vi "genRVCtraj.vi"() -> ()   [LabVIEW 2016]
uses:
  <vilib>/Math Plots/3D Math Plots/3D Scatter/3D Scatter XCtrl/3D Scatter.xctl
  <vilib>/Analysis/1siggen.llb/Ramp Pattern by Samples.vi
  <vilib>/Utility/file.llb/Read Delimited Spreadsheet (DBL).vi
  Subsystems/Global Variables.vi
  <vilib>/Math Plots/3D Math Plots/3D Scatter/3D Scatter Datatype/Public/Plot Helper (Vector).vi
  <vilib>/Math Plots/3D Math Plots/3D Scatter/3D Scatter Datatype/3D Scatter Datatype.lvclass
  <vilib>/gmath/NI_Gmath.lvlib
  <vilib>/Analysis/NI_AALBase.lvlib
panel:
  out "DH Params":cluster{"d_DH":dbl[][], "ty":dbl[][]}
  out "J3 Array":dbl[](array[numeric])
  out "J2 Array":dbl[](array[numeric])
  out "J1 Array":dbl[](array[numeric])
  in  "offsetZ":dbl
  in  "offsetX":dbl
  in  "offsetY":dbl
  out "size(s)":i32
  out "zVisTraj":dbl[](array[numeric]) format="%_6g"
  out "yVisTraj":dbl[](array[numeric]) format="%_6g"
  out "xVisTraj":dbl[](array[numeric]) format="%_6g"
  out "Groove Plot":refnum<class "3D Plot Datatype.lvclass">[](xcontrol)
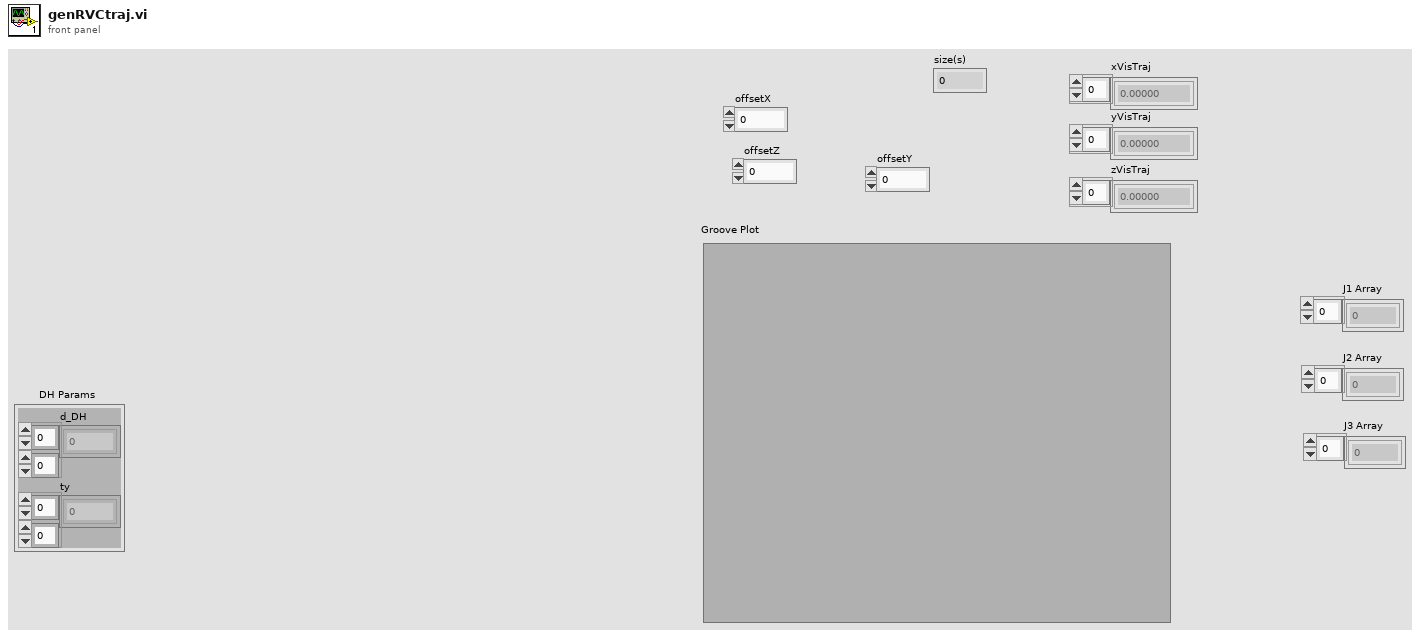
[diagram p1: front panel]
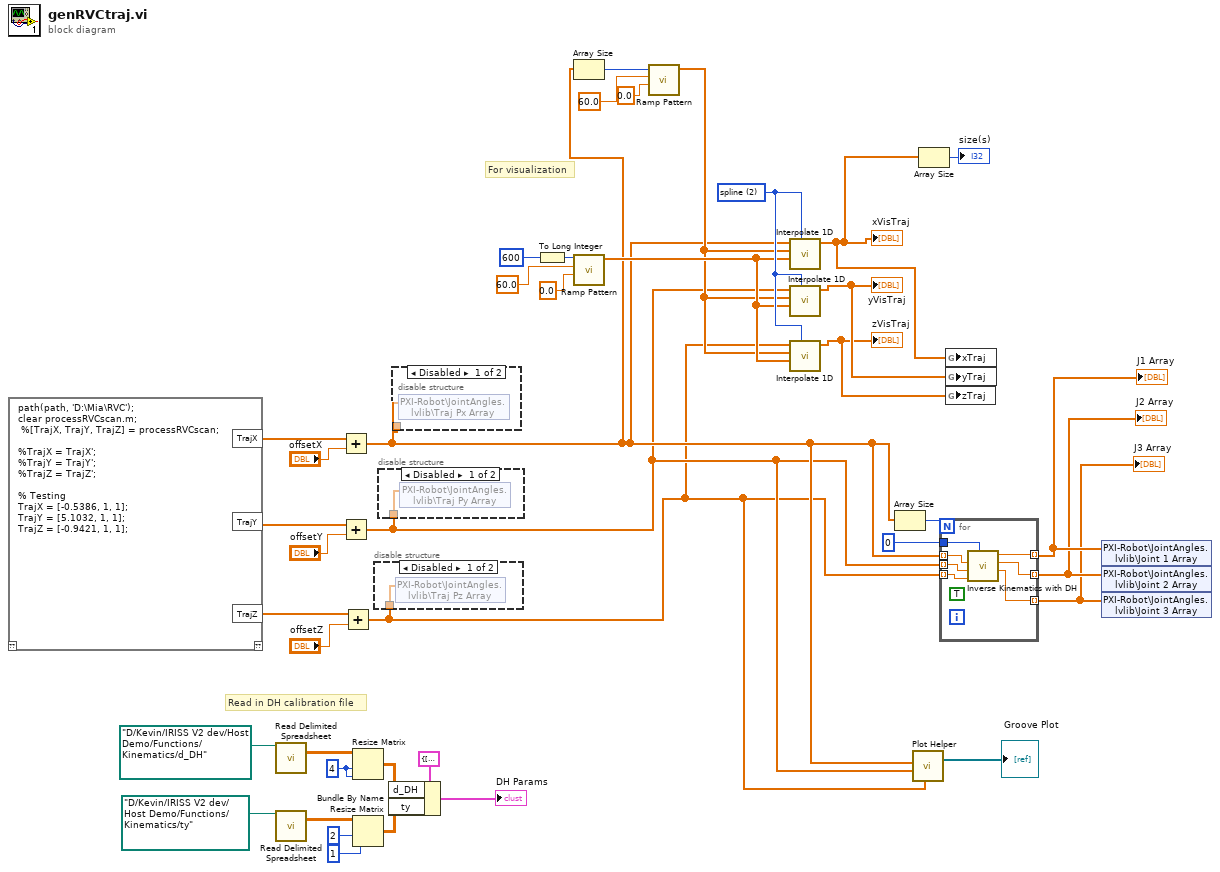
[diagram p0: block diagram]
diagram:
  w9 = 4 ("number of rows")
  w40 = 2 items=["nearest", "linear", "spline", "cubic Hermite", "Lagrange"] ("method")
  # "Read in DH calibration file"
  # "For visualization"
  n1 = script code="path(path, 'D:\\Mia\\RVC'); \nclear processRVCscan.m; \n %[TrajX, TrajY, TrajZ] = processRVCscan; \n\n%TrajX = TrajX'; \n%TrajY = TrajY'; \n%TrajZ = TrajZ'; \n\n% Testing \nTrajX = [-0.5386, 1, 1]; \nTrajY = [5.1032, 1, 1]; \nTrajZ = [-0.9421, 1, 1];"() -> ("TrajX"=w19:dbl[], "TrajY"=w18:dbl[], "TrajZ"=w16:dbl[])  [unwired: 1 in, 1 out]
  n2 = call-poly <vilib>:"Read Delimited Spreadsheet.vi"("file path (dialog if empty)"=path "D:/Kevin/IRISS V2 dev/Host Demo/Functions/Kinematics/d_DH" ("file path (use dialog)")) -> ("all rows"=w10:dbl[][])  [unwired: 9 in, 5 out]
  n3 = call-poly <vilib>:"Read Delimited Spreadsheet.vi"("file path (dialog if empty)"=path "D:/Kevin/IRISS V2 dev/Host Demo/Functions/Kinematics/ty" ("file path (use dialog)")) -> ("all rows"=w8:dbl[][])  [unwired: 9 in, 5 out]
  n4 = Add(x=w19, y="offsetX") -> (x+y=w20:dbl[])
  n5 = Add(x=w18, y="offsetY") -> (x+y=w17:dbl[])
  n6 = Add(x=w16, y="offsetZ") -> (x+y=w15:dbl[])
  n7 = Resize Matrix(1:w9, 2:w9, 4:w10) -> (0:w4:dbl[][])
  n8 = Resize Matrix(1:1 ("number of columns"), 2:2 ("number of rows"), 4:w8) -> (0:w3:dbl[][])
  n9 = disable-structure shown="Disabled" {
    disable-tunnel: w15 -> [w41 _]
    frame Disabled {
      n10 = shared-variable "PXI-Robot\\JointAngles.lvlib\\Traj Pz Array"(w41) -> ()  [unwired: 1 in, 1 out]
    }
    frame Enabled {
    }
  }
  n11 = disable-structure shown="Disabled" {
    disable-tunnel: w17 -> [w42 _]
    frame Disabled {
      n12 = shared-variable "PXI-Robot\\JointAngles.lvlib\\Traj Py Array"(w42) -> ()  [unwired: 1 in, 1 out]
    }
    frame Enabled {
    }
  }
  n13 = Bundle By Name(cluster=cluster{"d_DH":dbl[][], "ty":dbl[][]} {"d_DH"=[[0.0, -0.04858099004841317, 1.1971672750675049, 0.0], [0.0, -1.576475511297109, 0.0, 0.0], [-0.3552491783526254, 0.0, -1.1064589410656984, 0.2058446720735121], [-1.0573457532495087, 1.0278049025155533, 0.011917110633363169, -0.004023577880993236]], "ty"=[[0.04320445582455471], [0.011728642746432275]]} ("input cluster"), "d_DH"=w4, "ty"=w3) -> (→"DH Params":cluster{"d_DH":dbl[][], "ty":dbl[][]})
  n14 = disable-structure shown="Disabled" {
    disable-tunnel: w20 -> [w43 _]
    frame Disabled {
      n15 = shared-variable "PXI-Robot\\JointAngles.lvlib\\Traj Px Array"(w43) -> ()  [unwired: 1 in, 1 out]
    }
    frame Enabled {
    }
  }
  n16 = To Long Integer(number=600) -> (32bit integer=w39:i32)
  n17 = Array Size(array=w20) -> (size(s)=w33:i32)
  n18 = call-poly <vilib>:"Ramp Pattern.vi"("start"=0.0, "end"=60.0, "samples"=w39) -> ("Ramp Pattern"=w37:dbl[])  [unwired: 7 in, 1 out]
  n19 = call-poly <vilib>:"Ramp Pattern.vi"("start"=0.0, "end"=60.0, "samples"=w33) -> ("Ramp Pattern"=w32:dbl[])  [unwired: 7 in, 1 out]
  n20 = call <vilib>:"Interpolate 1D.vi"("method"=w40, "xi"=w37, "X"=w32, "Y"=w20) -> ("yi"=w29:dbl[])  [unwired: 5 in, 2 out]
  "xVisTraj" <- w29
  n21 = call <vilib>:"Interpolate 1D.vi"("method"=w40, "xi"=w37, "X"=w32, "Y"=w17) -> ("yi"=w28:dbl[])  [unwired: 5 in, 2 out]
  "yVisTraj" <- w28
  n22 = call <vilib>:"Interpolate 1D.vi"("method"=w40, "xi"=w37, "X"=w32, "Y"=w15) -> ("yi"=w27:dbl[])  [unwired: 5 in, 2 out]
  "zVisTraj" <- w27
  n23 = Array Size(array=w20) -> (size(s)=w26:i32)
  n24 = call-poly <vilib>:"Plot Helper.vi"("z vector"=w15, "y vector"=w17, "x vector"=w20) -> ("3D Plot lvclass Array out"=→"Groove Plot":refnum<class "3D Plot Datatype.lvclass">[])  [unwired: 3 in, 5 out]
  n25 = Array Size(array=w29) -> (size(s)=→"size(s)":i32)
  n26 = for {
    N: w26 -> [_]
    tunnel: 0 ("Arm ID Ind") -> [w50]
    tunnel: w20 -> [w49] mode=indexing
    tunnel: w17 -> [w48] mode=indexing
    tunnel: w15 -> [w47] mode=indexing
    tunnel: [w44] -> w14 mode=indexing
    tunnel: [w45] -> w13 mode=indexing
    tunnel: [w46] -> w12 mode=indexing
    (unwired) TRUE ("isToolTipInsideEye")
    n27 = call "Inverse Kinematics with DH.vi"("armID"=w50, "z"=w47, "y"=w48, "x"=w49) -> ("j3"=w46:dbl, "j2"=w45:dbl, "j1"=w44:dbl)  [unwired: 5 in]
  }
  "J1 Array" <- w14
  "J2 Array" <- w13
  "J3 Array" <- w12
  n28 = global write "Global Variables.vi" "xTraj"(w29) -> ()
  n29 = global write "Global Variables.vi" "yTraj"(w28) -> ()
  n30 = global write "Global Variables.vi" "zTraj"(w27) -> ()
  n31 = shared-variable "PXI-Robot\\JointAngles.lvlib\\Joint 1 Array"(w14) -> ()  [unwired: 1 in, 1 out]
  n32 = shared-variable "PXI-Robot\\JointAngles.lvlib\\Joint 2 Array"(w13) -> ()  [unwired: 1 in, 1 out]
  n33 = shared-variable "PXI-Robot\\JointAngles.lvlib\\Joint 3 Array"(w12) -> ()  [unwired: 1 in, 1 out]
